vi "VC Configure Hardware.vi"(8 "error in (no error)":errorcluster, 10 "input cluster":T1, 11 "Hardware Resources in":T2) -> (0 "error out":errorcluster, 3 "Hardware Resources out":T2)   [LabVIEW 2020, in "Valve Control.lvlib"]
doc: "Configure the hardware."
uses:
  Valve Control.lvlib
  AM Configuration.ctl
  support/Message Queue/Message Cluster.ctl
  support/Message Queue/All Message Queues.ctl
  support/Message Queue/Message Queue.lvlib
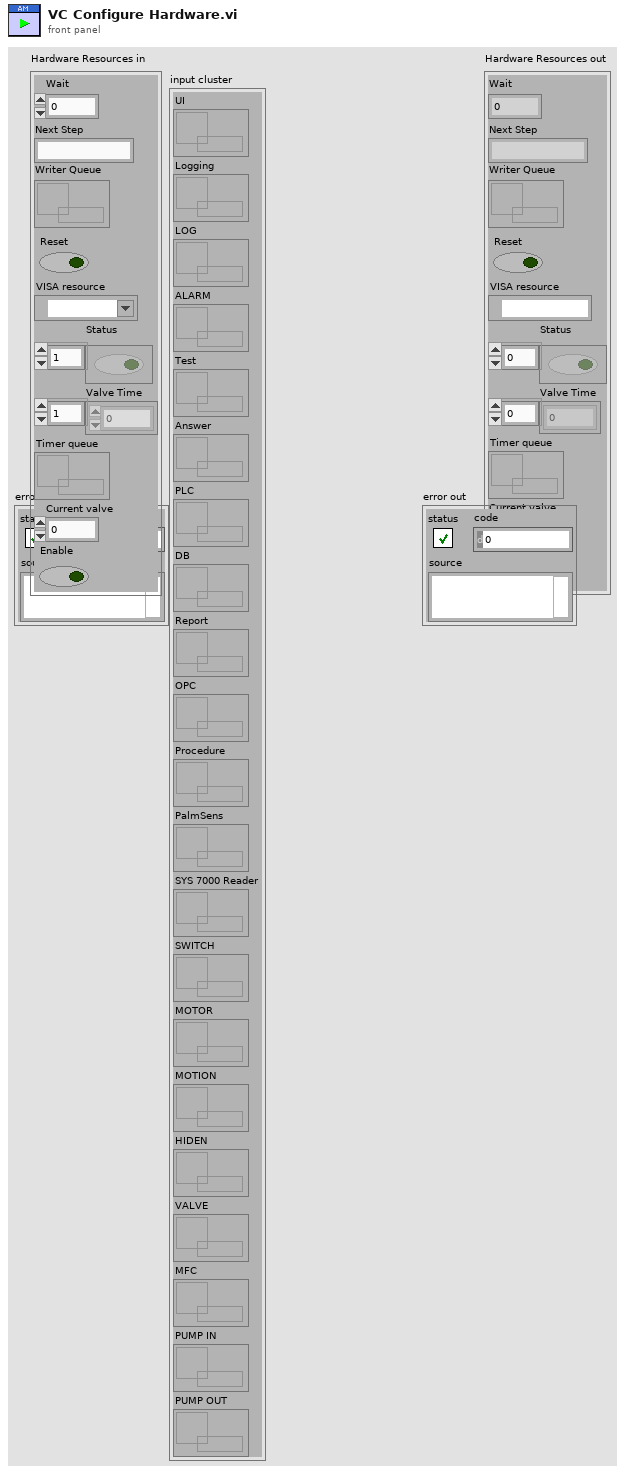
[diagram p1: front panel]
types:
  T1 = typedef "Message Queue.lvlib/All Message Queues.ctl" = cluster{"UI":refnum<queue>, "Logging":refnum<queue>, "LOG":refnum<queue>, "ALARM":refnum<queue>, "Test":refnum<queue>, "Answer":refnum<queue>, "PLC":refnum<queue>, "DB":refnum<queue>, "Report":refnum<queue>, "OPC":refnum<queue>, "Procedure":refnum<queue>, "PalmSens":refnum<queue>, "SYS 7000 Reader":refnum<queue>, "SWITCH":refnum<queue>, "MOTOR":refnum<queue>, "MOTION":refnum<queue>, "HIDEN":refnum<queue>, "VALVE":refnum<queue>, "MFC":refnum<queue>, "PUMP IN":refnum<queue>, "PUMP OUT":refnum<queue>}
  T2 = typedef "Valve Control.lvlib/AM Configuration.ctl" = cluster{"Wait":dbl, "Next Step":string, "Writer Queue":refnum<queue>, "Reset":bool, "VISA resource":refnum<visa-resource-name>, "Status":bool[], "Valve Time":dbl[], "Timer queue":refnum<queue>, "Current valve":i32, "Enable":bool}
  T3 = cluster{"Type CMD":string, "Mode CMD":string, "Main CMD":string}
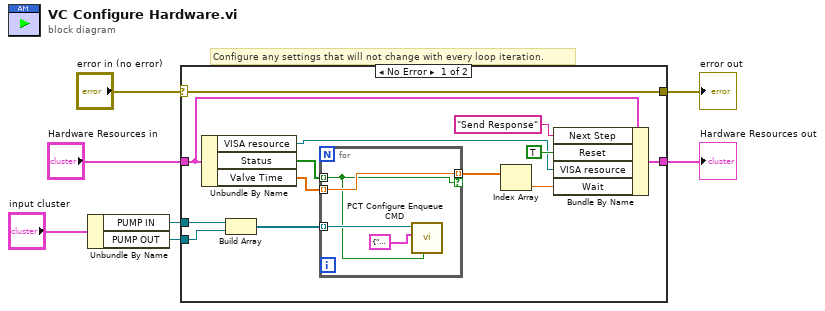
[diagram p0: block diagram]
diagram:
  # "Configure any settings that will not change with every loop iteration."
  n1 = Unbundle By Name("input cluster") -> ("PUMP IN"=w2:refnum<queue>, "PUMP OUT"=w1:refnum<queue>)
  n2 = case shown="No Error" "error in (no error)" {
    selector: "error in (no error)" -> [w20 w25]
    tunnel: [w20 w25] -> w6
    tunnel: "Hardware Resources in" -> [w16 w26]
    tunnel: [w19 w26] -> w4
    tunnel: w2 -> [w11 _]
    tunnel: w1 -> [w10 _]
    frame No Error {
      n3 = Unbundle By Name(w16) -> ("VISA resource"=w8:refnum<visa-resource-name>, "Status"=w15:bool[], "Valve Time"=w14:dbl[])
      n4 = Build Array(w11, w10) -> (w9:refnum<queue>[])
      n5 = for {
        tunnel: w15 -> [w21] mode=indexing
        tunnel: w14 -> [w24] mode=indexing
        tunnel: [w24] -> w13 mode=indexing if=w21
        tunnel: w9 -> [w22] mode=indexing
        n6 = call "PCT Configure Enqueue CMD.vi"("Parameter Data"=w21, "CMD"=T3 {"Type CMD"="Run", "Mode CMD"="", "Main CMD"="Action-Status"}, "CMD Queue in"=w22) -> ()  [unwired: 6 in, 3 out]
      }
      n7 = Index Array(array=w13) -> (element=w12:dbl)  [unwired: 1 in]
      n8 = Bundle By Name(cluster=w16, "Next Step"="Send Response", "Reset"=TRUE, "VISA resource"=w8, "Wait"=w12) -> (w19:T2)
    }
    frame Error {
    }
  }
  "Hardware Resources out" <- w4
  "error out" <- w6
